vi "MedianFilter_Execute.vi"(9 "Enable":bool=TRUE, 10 "Samples":i32, 11 "Input Value":dbl) -> (1 "MedianValue":dbl, 3 "Out MEDIAN_FILTER":T1 {"ValueBuffer" format="%13.5g"})   [LabVIEW 2019, in "Trajectory_Library.lvlib"]
doc: "Convience, single call, LabVIEW function. Creates and calculates the moving-window median for the next value of the input stream.\nThe optional enable parameter bypasses the filter calculation when \"enabled\" is false. When enabled is \"false\" the internal buffer is continually filled with the current input value.\n\nThis implements a moving-window median filter. Useful for reducing measurement noise, especially with processes that generate occasional, extreme outliers (such as values from vision processing, LIDAR, or ultrasonic sensors).\n\nInputs:\n - Input Value -- The next input value. \n - samples -- The number of samples in the moving window.\n - enable -- Perform the filter calcuation when True. When False, output the input value unchanged. (Default=True)\n\nOutputs:\n - Out Median Filter -- Updated median filter data structure\n - Median Value -- The median of the moving window, updated to include the next value.."
uses:
  Trajectory_Library.lvlib
  MEDIAN_FILTER.ctl
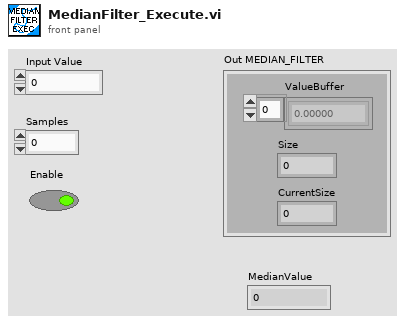
[diagram p1: front panel]
types:
  T1 = typedef "Trajectory_Library.lvlib/MEDIAN_FILTER.ctl" = cluster{"ValueBuffer":dbl[], "Size":i32, "CurrentSize":i32}
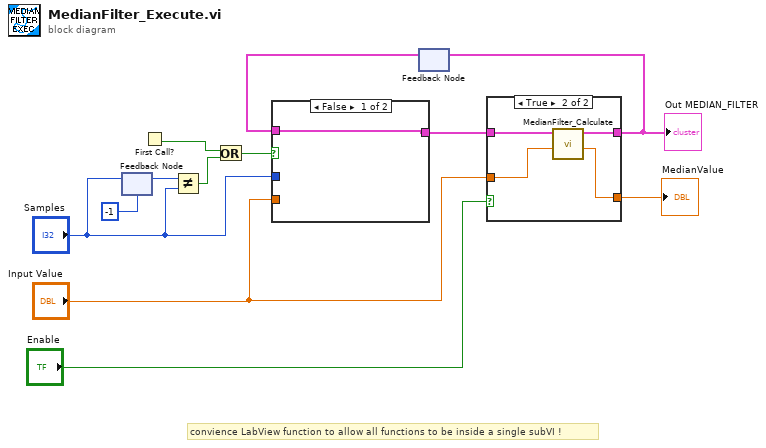
[diagram p0: block diagram]
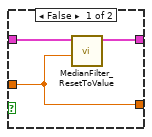
[diagram p2: hidden frame]
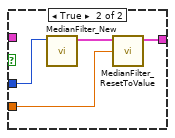
[diagram p3: hidden frame]
diagram:
  # "convience LabView function to allow all functions to be inside a single subVI !"
  n1 = feedback-in #1("Samples") -> ()
  n2 = feedback #1(-1 ("Samples")) -> (w6:i32)
  n3 = First Call?() -> (First Call?: T/F=w3:bool)
  n4 = Not Equal?(x=w6, y="Samples") -> (x != y?=w7:bool)
  n5 = Or(x=w3, y=w7) -> (x .or. y?=w8:bool)
  n6 = feedback #2() -> (w10:T1)  [unwired: 1 in]
  n7 = case shown="False" w8 {
    tunnel: w10 -> [w13 _]
    tunnel: "Samples" -> [_ w16]
    tunnel: "Input Value" -> [_ w15]
    tunnel: [w13 w14] -> w2
    frame False {
    }
    frame True {
      n8 = call "MedianFilter_New.vi"("Samples"=w16) -> ("MEDIAN_FILTER"=w17:T1)  [unwired: 10 in]
      n9 = call "MedianFilter_ResetToValue.vi"("Value"=w15, "In MEDIAN_FILTER"=w17) -> ("Out MEDIAN_FILTER"=w14:T1)  [unwired: 9 in]
    }
  }
  n10 = case shown="True" "Enable" {
    tunnel: w2 -> [w20 w24]
    tunnel: [w19 w23] -> w9
    tunnel: "Input Value" -> [w18 w22]
    tunnel: [w18 w21] -> w11
    frame False {
      n11 = call "MedianFilter_ResetToValue.vi"("Value"=w18, "In MEDIAN_FILTER"=w20) -> ("Out MEDIAN_FILTER"=w19:T1)  [unwired: 9 in]
    }
    frame True {
      n12 = call "MedianFilter_Calculate.vi"("Input Value"=w22, "In MEDIAN_FILTER"=w24) -> ("MedianValue"=w21:dbl, "Out MEDIAN_FILTER"=w23:T1)  [unwired: 8 in]
    }
  }
  "Out MEDIAN_FILTER" <- w9
  "MedianValue" <- w11
  n13 = feedback-in #2(w9) -> ()
